vi "AR-Predict.vi"(6 "thickness":i32=100, 7 "width":i32=1000, 8 "AR coeff":dbl[](array[numeric]), 9 "p":dbl=13.0, 11 "filtered signal":dbl[](array[numeric])) -> (2 "predicted signal":dbl[](array[numeric]))   [LabVIEW 2017]
uses:
  <vilib>/Analysis/baseanly.llb/Real Dot Product.vi
  <vilib>/Analysis/NI_AALBase.lvlib
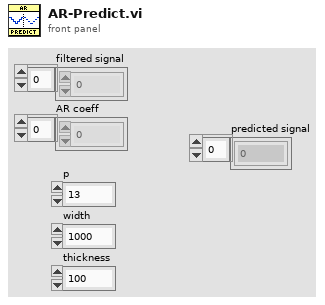
[diagram p1: front panel]
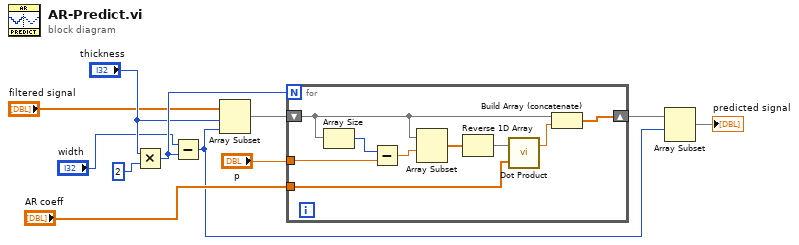
[diagram p0: block diagram]
diagram:
  n1 = Multiply(x="thickness", y=2) -> (x*y=w11:i32)
  n2 = Subtract(x="width", y=w11) -> (x-y=w1:i32)
  n3 = Array Subset(array="filtered signal", index="thickness", length=w1) -> (w10:dbl[])
  n4 = for {
    N: w11 -> [_]
    shift-right: [w13] -> w4
    shift-left: w10 -> [w12]
    tunnel: "AR coeff" -> [w20]
    tunnel: "p" -> [w18]
    n5 = Array Size(array=w12) -> (size(s)=w19:i32)
    n6 = Subtract(x=w19, y=w18) -> (x-y=w17:dbl)
    n7 = Array Subset(array=w12, index=w17) -> (w16:dbl[])  [unwired: 1 in]
    n8 = Reverse 1D Array(array=w16) -> (reversed array=w15:dbl[])
    n9 = call-poly <vilib>:"Dot Product.vi"("Y Vector"=w20, "X Vector"=w15) -> ("X * Y"=w14:dbl)  [unwired: 1 out]
    n10 = Build Array (concatenate)(w12, w14) -> (w13:dbl[])
  }
  n11 = Array Subset(array=w4, index=w1) -> (→"predicted signal":dbl[])  [unwired: 1 in]
